vi "Is VI Locked or Open.vi"(8 "Error In":errorcluster, 11 "VI Info":T1) -> (0 "Error Out":errorcluster, 3 "Locked or Open?":bool)   [LabVIEW 2020, in "Peek Window.lvlib"]
uses:
  Peek Window.lvlib
  dc01a00f-243c-4d6c-abee-c709533ad71c.vi
  Open Diagram Argument--cluster.ctl
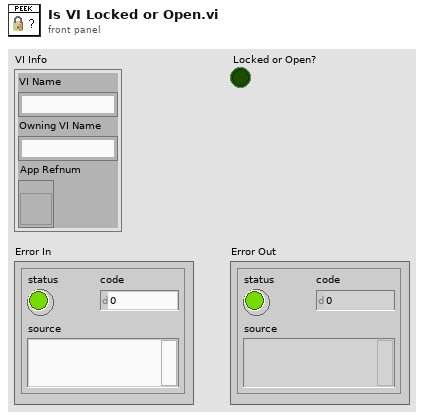
[diagram p1: front panel]
types:
  T1 = typedef "Peek Window.lvlib/Open Diagram Argument--cluster.ctl" = cluster{"VI Name":string, "Owning VI Name":string, "App Refnum":refnum<vi>}
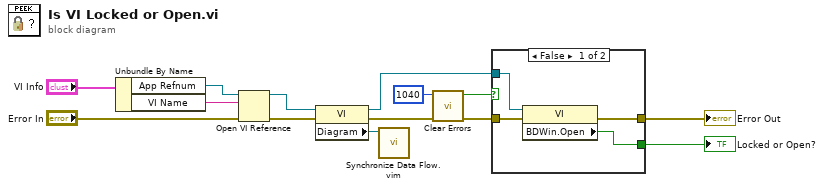
[diagram p0: block diagram]
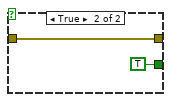
[diagram p2: hidden frame]
diagram:
  n1 = Unbundle By Name("VI Info") -> ("App Refnum"=w2:refnum<vi>, "VI Name"=w1:string)
  n2 = Open VI Reference(application reference (local)=w2, vi path=w1, error in (no error)="Error In") -> (vi reference=w13:refnum<vi>, error out=w12:errorcluster)  [unwired: 3 in]
  n3 = property class="VI"(reference=w13, error in=w12) -> (reference out=w5:refnum<vi>, error out=w10:errorcluster, "Diagram"=w4:refnum<vi>)
  n4 = call "Synchronize Data Flow.vim"("input 1"=w4) -> ()  [unwired: 3 in, 4 out]
  n5 = call <vilib>:"Clear Errors.vi"("error in (no error)"=w10, "specific error code to clear (0: all)"=1040) -> ("error out"=w8:errorcluster, "specific error cleared?"=w9:bool)  [unwired: 4 in]
  n6 = case shown="False" w9 {
    tunnel: w8 -> [w18 w20]
    tunnel: [w17 w20] -> w7
    tunnel: [w15 TRUE ("Locked or Open?")] -> w6
    tunnel: w5 -> [w16 _]
    frame False {
      n7 = property class="VI"(reference=w16, error in=w18) -> (error out=w17:errorcluster, "BDWin.Open"=w15:bool)  [unwired: 1 out]
    }
    frame True {
    }
  }
  "Error Out" <- w7
  "Locked or Open?" <- w6
